vi "Send String.vi"(6 "error in (no error)":errorcluster, 8 "Bus In":refnum<class "Bus.lvclass">, 9 "String Init In":refnum<class "String Init.lvclass">) -> (0 "error out":errorcluster, 2 "Bus Out":refnum<class "Bus.lvclass">, 3 "String Init out":refnum<class "String Init.lvclass">)   [LabVIEW 2018, in "String Init.lvclass"]
doc: "String init.lvclass:Send String.vi\n\nThis VI is used to send a string through the bus.\n\nInstrument Communication Module Version 1.0\nOctober, 2020 Original Code Consulting Davita Bird\n www.originalcode.com"
uses:
  String Init.lvclass
  Bus/Bus.lvclass
  String Init.lvclass/String Init.ctl
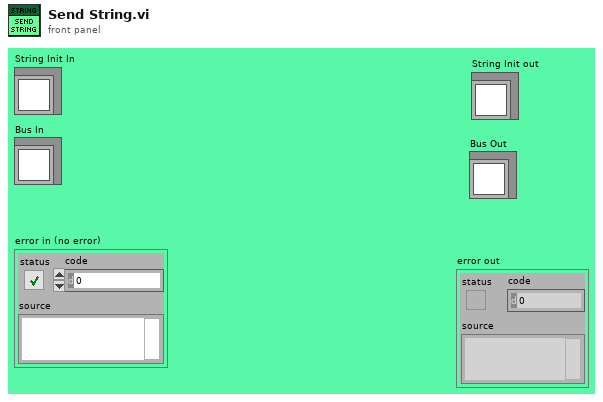
[diagram p1: front panel]
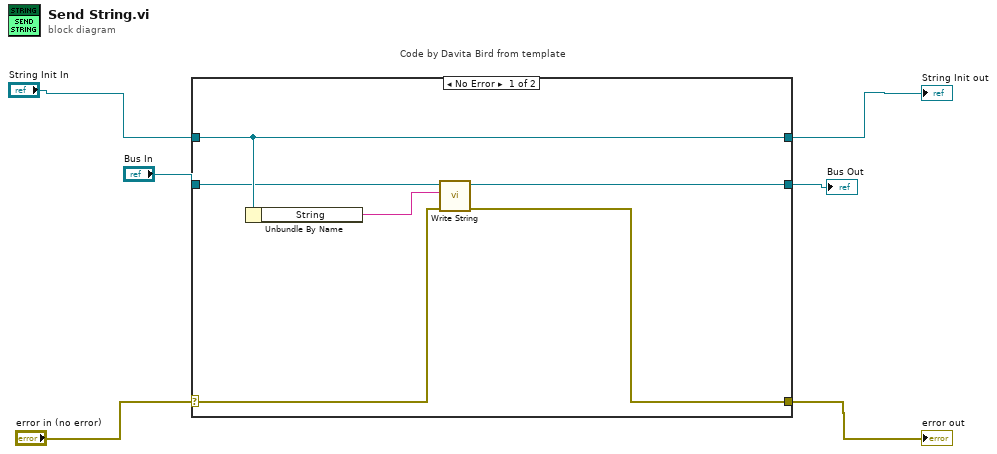
[diagram p0: block diagram]
diagram:
  n1 = case "Code by Davita Bird from template" shown="No Error" "error in (no error)" {
    selector: "error in (no error)" -> [w9 w15]
    tunnel: [w7 w15] -> w1
    tunnel: [w12 w14] -> w5
    tunnel: "String Init In" -> [w12 w14]
    tunnel: [w8 w13] -> w3
    tunnel: "Bus In" -> [w11 w13]
    frame No Error {
      n2 = Unbundle By Name(w12) -> ("String"=w10:string)
      n3 = call-dynamic "Write String.vi"("error in (no error)"=w9, "String"=w10, "Bus in"=w11) -> ("error out"=w7:errorcluster, "Bus out"=w8:refnum<class "Bus.lvclass">)  [unwired: 7 in]
    }
    frame Error {
    }
  }
  "error out" <- w1
  "String Init out" <- w5
  "Bus Out" <- w3
